vi "SV Continuous Swept-Sine Harmonic Waveform.vi"(0 "scaled signals [EU]":waveform(dbl)[](array[waveform]), 2 "reset? (F)":bool, 5 "harmonic":i32=1, 11 "error in (no error)":errorcluster, 13 "zero delay? (F)":bool) -> (4 "scaled signals out [EU]":waveform(dbl)[](array[waveform]), 6 "harmonic waveforms":waveform(dbl)[](array[waveform]), 8 "residue waveforms":waveform(dbl)[](array[waveform]), 15 "error out":errorcluster)   [LabVIEW 2017, in "SoundVib_ContSweptSine.lvlib"]
doc: "Extracts the time-domain waveform and residue waveform from one specific harmonic by performing a continuous swept-sine measurement."
uses:
  <vilib>/addons/Sound and Vibration/svt_Continuous Swept Sine/SoundVib_ContSweptSine.lvlib
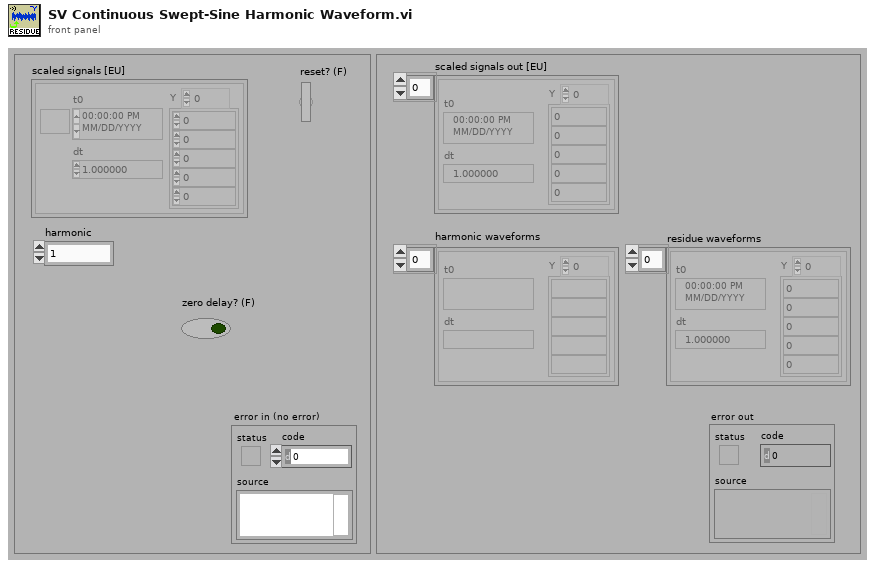
[diagram p1: front panel]
types:
  T1 = typedef "svc_Resampled Channel Info.ctl" = cluster{"channel name":string, "description":string, " channel info":T2}
  T2 = typedef "svc_Channel Info.ctl" = cluster{"sensor sensitivity":dbl, "engineering units":T3, "dB reference":dbl, "custom label":string, "weighting filter":T4, "pregain":dbl}
  T3 = typedef "svc_Engineering Units Text Ring.ctl" = u16
  T4 = typedef "svc_Weighting Filter Text Ring.ctl" = u16
  T5 = typedef "OAT Position Info.ctl" = cluster{"positions [s]":dbl[], "samples/rev":dbl}
  T6 = typedef "SoundVib_Generation.lvlib/sv_Chirp Settings.ctl" = cluster{"amplitude":dbl, "frequency range":cluster{"start (Hz)":dbl, "stop (Hz)":dbl, "frequency spacing":enum16{"Linear", "Logarithmic"}}, "sampling info":cluster{"Fs":dbl, "chirp duration [s]":dbl}, "initial states":cluster{"frequency [Hz]":dbl, "phase [rad]":dbl, "elapsed time [s]":dbl}, "frequency slope":dbl, "maximum harmonic":i32, "prefix len [samples]":cluster{"integer":u32, "fractional":dbl}}
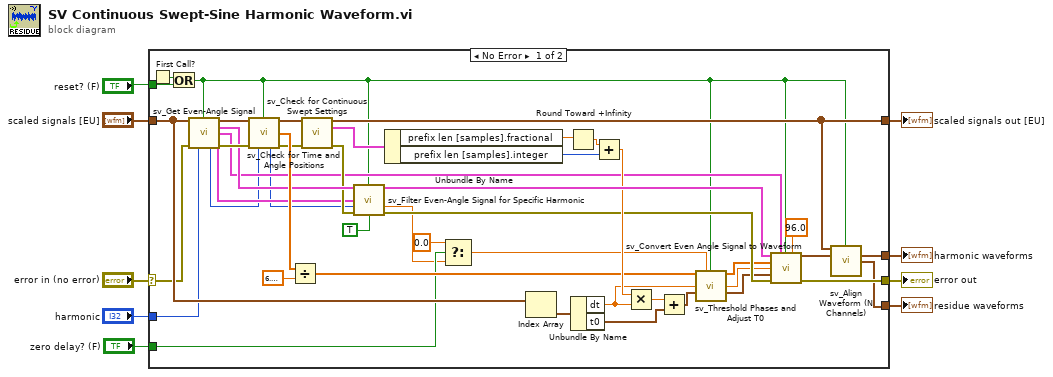
[diagram p0: block diagram]
diagram:
  n1 = case shown="No Error" "error in (no error)" {
    selector: "error in (no error)" -> [w45 w56]
    tunnel: [w35 w56] -> w8
    tunnel: [w30 _] -> w7
    tunnel: "scaled signals [EU]" -> [w47 w55]
    tunnel: [w31 w55] -> w5
    tunnel: "harmonic" -> [w11 _]
    tunnel: [w13 _] -> w3
    tunnel: "zero delay? (F)" -> [w21 _]
    tunnel: "reset? (F)" -> [w15 _]
    frame No Error {
      n2 = First Call?() -> (First Call?: T/F=w16:bool)
      n3 = Or(x=w16, y=w15) -> (x .or. y?=w14:bool)
      n4 = call <vilib>:"sv_Get Even-Angle Signal.vi"("data to process"=w47, "reset?"=w14, "error in (no error)"=w45, "maximum harmonic"=w11) -> ("data to process out"=w53:waveform(dbl)[], "even-angle signals"=w43:cluster{"r0":dbl, "dr":dbl, "Y":dbl[]}[], "even-angle channel info"=w22:T1[], "even-angle position info"=w29:T5, "actual maximum harmonic"=w10:i32, "error out"=w44:errorcluster)  [unwired: 6 in]
      n5 = call <vilib>:"sv_Check for Time and Angle Positions.vi"("data to process"=w53, "reset?"=w14, "error in (no error)"=w44, "harmonic"=w10) -> ("data to process out"=w49:waveform(dbl)[], "phase array [rad]"=w52:dbl[], "actual harmonic"=w12:i32, "error out"=w48:errorcluster)  [unwired: 6 in, 2 out]
      n6 = Divide(x=w52, y=6.283185307179586) -> (x/y=w28:dbl[])
      n7 = call <vilib>:"sv_Check for Continuous Swept Settings.vi"("data to process"=w49, "error in (no error)"=w48) -> ("data to process out"=w31:waveform(dbl)[], "chirp settings"=w46:T6, "error out"=w34:errorcluster)  [unwired: 11 in]
      n8 = call <vilib>:"sv_Filter Even-Angle Signal for Specific Harmonic.vi"("even-angle signals"=w43, "reset?"=w14, "even-angle position info"=w29, "specific harmonic"=w12, "error in (no error)"=w34, "zero delay? (F)"=TRUE) -> ("even-angle signals out"=w42:cluster{"r0":dbl, "dr":dbl, "Y":dbl[]}[], "phase delay [1/cycle]"=w20:dbl, "error out"=w33:errorcluster)  [unwired: 6 in, 1 out]
      n9 = Unbundle By Name(w46) -> ("prefix len [samples].fractional"=w41:dbl, "prefix len [samples].integer"=w39:u32)
      n10 = Select(t=0.0, s=w21, f=w20) -> (s? t:f=w19:dbl)
      n11 = Index Array(array=w47) -> (element=w51:waveform(dbl))  [unwired: 1 in]
      n12 = Round Toward +Infinity(x=w41) -> (ceil(x): smallest int >= x=w40:dbl)
      n13 = Unbundle By Name(w51) -> ("dt"=w27:dbl, "t0"=w36:timestamp)
      n14 = Add(x=w40, y=w39) -> (x+y=w38:dbl)
      n15 = Multiply(x=w38, y=w27) -> (x*y=w37:dbl)
      n16 = Add(x=w37, y=w36) -> (x+y=w25:timestamp)
      n17 = call <vilib>:"sv_Threshold Phases and Adjust T0.vi"("Phases [1/cycle]"=w28, "phase delay [1/cycle]"=w19, "reset?"=w14, "dt"=w27, "t0"=w25) -> ("Phases [1/cycle]"=w23:dbl[], "dt out"=w26:dbl, "t0 out"=w24:timestamp)  [unwired: 8 in]
      n18 = call <vilib>:"sv_Convert Even Angle Signal to Waveform.vi"("even-angle signals"=w42, "even-angle channel info"=w22, "reset? (F)"=w14, "stopband attenuation [dB]"=96.0, "new sample phase"=w23, "new dt"=w26, "new t0"=w24, "error in (no error)"=w33) -> ("Waveform"=w32:waveform(dbl)[], "error out"=w35:errorcluster)  [unwired: 6 in]
      n19 = call <vilib>:"sv_Align Waveform (N Channels).vi"("waveforms"=w31, "reset?"=w14, "filtered waveforms"=w32) -> ("filtered waveforms out"=w30:waveform(dbl)[], "residue waveforms"=w13:waveform(dbl)[])  [unwired: 10 in, 1 out]
    }
    frame Error {
    }
  }
  "error out" <- w8
  "harmonic waveforms" <- w7
  "scaled signals out [EU]" <- w5
  "residue waveforms" <- w3
